vi "NIIE_Undo_Replay Data from History.vi"(8 "Error":errorcluster, 10 "Data":string[](array[string]), 11 "Data":T1={"Class"={"Ants"=refnum, "Layer"=refnum, "Templates"=refnum, "Icon"=refnum, "Glyph"=refnum, "Settings"=refnum, "Tools"=refnum}, "Ref"={"Add Layer"=refnum, "Remove Layer"=refnum, "Line Text"=[], "Body Text Spec"=refnum, "DNL_Font"=refnum, "glyph path str"=refnum, "templates path str"=refnum, "Arrow Up"=refnum, "Arrow Down"=refnum, "IE VI Ref"=refnum, "Glyphs tree"=refnum, "Templates tree"=refnum, "Layer Icon Text"=refnum, "Layer Template"=refnum, "Clipboard"=refnum, "BW icon in"=refnum, "Color icon in"=refnum, "Layer Clust"=refnum, "Body Text"=refnum, "DNL_Framework Templates"=refnum, "Search Templates"=refnum, "TextMarker"=refnum, "Tab Control"=refnum, "Search Glyphs"=refnum, "Line Color"=refnum, "DNL_Glyphs []"=refnum, "Fill Color"=refnum, "Tools"=refnum, "Glyphs tree"=refnum, "Icon"=refnum, "Preview"=refnum, "Ants"=refnum, "Terminals"=refnum, "menu reference"=refnum, "LayerNames"=[], "GlyphLoadAnimation"=refnum, "TemplateLoadAnimation"=refnum, "refreshGlyphs"=refnum, "refreshTemplates"=refnum}, "Support"={"AntsRect"={"left"=0, "top"=0, "right"=0, "bottom"=0}, "Mouse Move Coords"={"Horizontal"=0, "Vertical"=0}, "Mouse Down Coords"={"Horizontal"=0, "Vertical"=0}, "Temp Coord"={"Horizontal"=0, "Vertical"=0}, "Action"=enum."Default", "Edge Color"=4914962, "Fill Color"=16860, "Mouse Down?"=FALSE, "Draft Mode?"=FALSE, "Temp Icon"=bytes[3102], "CTRL Pressed"=FALSE, "Move Selection?"=FALSE, "AntsRect Orig"={"left"=0, "top"=0, "right"=0, "bottom"=0}, "Text"="", "TM Set?"=FALSE, "Mouse inside icon?"=FALSE, "Tool (old value)"=0, "Pencil Move Color"=0, "Swap Colors?"=FALSE, "Shift pressed?"=FALSE}}) -> (0 "Error Out":errorcluster, 3 "Data Out":T1={"Class"={"Ants"=refnum, "Layer"=refnum, "Templates"=refnum, "Icon"=refnum, "Glyph"=refnum, "Settings"=refnum, "Tools"=refnum}, "Ref"={"Add Layer"=refnum, "Remove Layer"=refnum, "Line Text"=[], "Body Text Spec"=refnum, "DNL_Font"=refnum, "glyph path str"=refnum, "templates path str"=refnum, "Arrow Up"=refnum, "Arrow Down"=refnum, "IE VI Ref"=refnum, "Glyphs tree"=refnum, "Templates tree"=refnum, "Layer Icon Text"=refnum, "Layer Template"=refnum, "Clipboard"=refnum, "BW icon in"=refnum, "Color icon in"=refnum, "Layer Clust"=refnum, "Body Text"=refnum, "DNL_Framework Templates"=refnum, "Search Templates"=refnum, "TextMarker"=refnum, "Tab Control"=refnum, "Search Glyphs"=refnum, "Line Color"=refnum, "DNL_Glyphs []"=refnum, "Fill Color"=refnum, "Tools"=refnum, "Glyphs tree"=refnum, "Icon"=refnum, "Preview"=refnum, "Ants"=refnum, "Terminals"=refnum, "menu reference"=refnum, "LayerNames"=[], "GlyphLoadAnimation"=refnum, "TemplateLoadAnimation"=refnum, "refreshGlyphs"=refnum, "refreshTemplates"=refnum}, "Support"={"AntsRect"={"left"=0, "top"=0, "right"=0, "bottom"=0}, "Mouse Move Coords"={"Horizontal"=0, "Vertical"=0}, "Mouse Down Coords"={"Horizontal"=0, "Vertical"=0}, "Temp Coord"={"Horizontal"=0, "Vertical"=0}, "Action"=enum."Default", "Edge Color"=4914962, "Fill Color"=16860, "Mouse Down?"=FALSE, "Draft Mode?"=FALSE, "Temp Icon"=bytes[3102], "CTRL Pressed"=FALSE, "Move Selection?"=FALSE, "AntsRect Orig"={"left"=0, "top"=0, "right"=0, "bottom"=0}, "Text"="", "TM Set?"=FALSE, "Mouse inside icon?"=FALSE, "Tool (old value)"=0, "Pencil Move Color"=0, "Swap Colors?"=FALSE, "Shift pressed?"=FALSE}})   [LabVIEW 2021]
uses:
  Controls/IE Data.ctl
  Class/Ants/Ants.lvclass
  Class/FakedArray/FakedArray.lvclass
  vi.lib/LabVIEW Icon API/lv_icon/Classes/Icon/Icon.lvclass
  Class/Icon Library/Glyph.lvclass
  Class/Settings/Settings.lvclass
  Class/Tools/Tools Paint.lvclass
  Controls/IE Classes.ctl
  Controls/References Cluster.ctl
  Controls/SupportClass.ctl
  <vilib>/Utility/miscctls.llb/LVPoint32TypeDef.ctl
  Controls/ENUM_SupportClass_Action.ctl
  vi.lib/LabVIEW Icon API/lv_icon/Controls/IEColor.ctl
  MB CORE/TypeDefs/Cluster_Layer Data.ctl
  MB CORE/TypeDefs/Cluster_Path&Icon.ctl
  MB CORE/TypeDefs/Cluster_BodyText.ctl
  vi.lib/LabVIEW Icon API/lv_icon/Controls/Font.ctl
  vi.lib/LabVIEW Icon API/lv_icon/Controls/Alignment.ctl
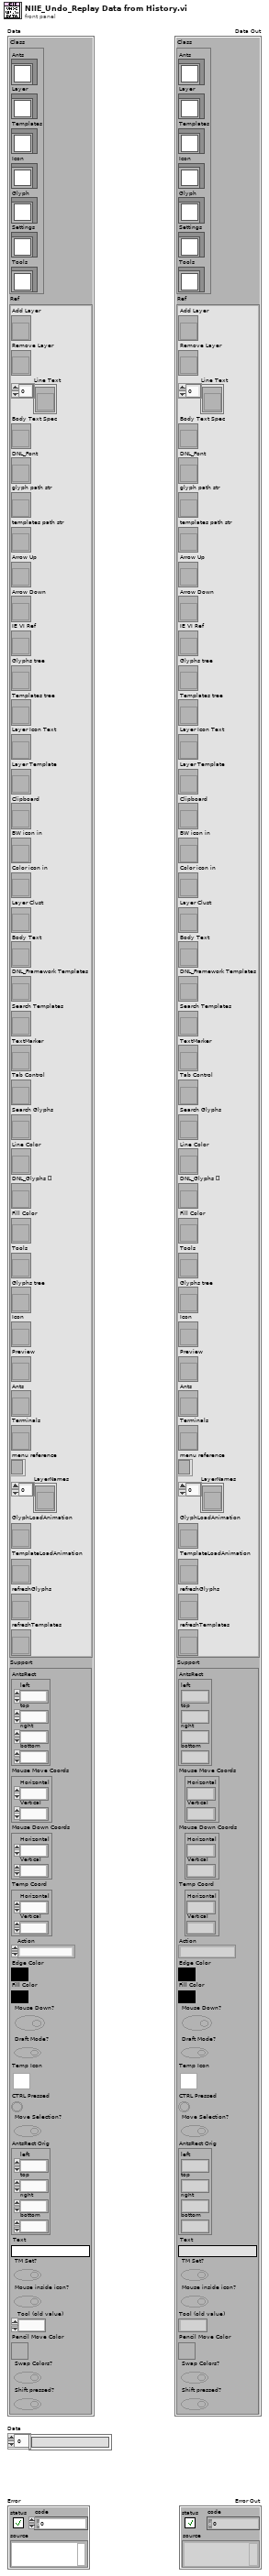
[diagram p1: front panel]
types:
  T1 = typedef "IE Data.ctl" = cluster{"Class":T2, "Ref":T3, "Support":T4}
  T2 = typedef "IE Classes.ctl" = cluster{"Ants":refnum<class "Ants.lvclass">, "Layer":refnum<class "FakedArray.lvclass">, "Templates":refnum<class "FakedArray.lvclass">, "Icon":refnum<class "Icon.lvclass">, "Glyph":refnum<class "Glyph.lvclass">, "Settings":refnum<class "Settings.lvclass">, "Tools":refnum<class "Tools Paint.lvclass">}
  T3 = typedef "References Cluster.ctl" = cluster{"Add Layer":refnum<vi>, "Remove Layer":refnum<vi>, "Line Text":refnum<vi>[], "Body Text Spec":refnum<vi>, "DNL_Font":refnum<vi>, "glyph path str":refnum<vi>, "templates path str":refnum<vi>, "Arrow Up":refnum<vi>, "Arrow Down":refnum<vi>, "IE VI Ref":refnum<vi>, "Glyphs tree":refnum<vi>, "Templates tree":refnum<vi>, "Layer Icon Text":refnum<vi>, "Layer Template":refnum<vi>, "Clipboard":refnum<vi>, "BW icon in":refnum<vi>, "Color icon in":refnum<vi>, "Layer Clust":refnum<vi>, "Body Text":refnum<vi>, "DNL_Framework Templates":refnum<vi>, "Search Templates":refnum<vi>, "TextMarker":refnum<vi>, "Tab Control":refnum<vi>, "Search Glyphs":refnum<vi>, "Line Color":refnum<vi>, "DNL_Glyphs []":refnum<vi>, "Fill Color":refnum<vi>, "Tools":refnum<vi>, "Glyphs tree":refnum<vi>, "Icon":refnum<vi>, "Preview":refnum<vi>, "Ants":refnum<vi>, "Terminals":refnum<vi>, "menu reference":refnum<k9>, "LayerNames":refnum<vi>[], "GlyphLoadAnimation":refnum<vi>, "TemplateLoadAnimation":refnum<vi>, "refreshGlyphs":refnum<vi>, "refreshTemplates":refnum<vi>}
  T4 = typedef "SupportClass.ctl" = cluster{"AntsRect":cluster{"left":i16, "top":i16, "right":i16, "bottom":i16}, "Mouse Move Coords":T5, "Mouse Down Coords":T5, "Temp Coord":T5, "Action":T6, "Edge Color":T7, "Fill Color":T7, "Mouse Down?":bool, "Draft Mode?":bool, "Temp Icon":picture, "CTRL Pressed":bool, "Move Selection?":bool, "AntsRect Orig":cluster{"left":i16, "top":i16, "right":i16, "bottom":i16}, "Text":string, "TM Set?":bool, "Mouse inside icon?":bool, "Tool (old value)":u32, "Pencil Move Color":u32, "Swap Colors?":bool, "Shift pressed?":bool}
  T5 = typedef "LVPoint32TypeDef.ctl" = cluster{"Horizontal":i32, "Vertical":i32}
  T6 = typedef "ENUM_SupportClass_Action.ctl" = enum16{"Default", "Move Selection", "Glyph Library", "Tool"}
  T7 = typedef "IEColor.ctl" = u32
  T8 = typedef "Cluster_BodyText.ctl" = cluster{"Line 1 text":string, "Line 2 text":string, "Line 3 text":string, "Line 4 text":string, "Line 1 color":u32, "Line 2 color":u32, "Line 3 color":u32, "Line 4 color":u32, "Body Text Spec":cluster{"Font":T9, "Alignment":T10, "Size":u8}, "Center text vertically":bool, "Capitalize Text":bool}
  T9 = typedef "Font.ctl" = string
  T10 = typedef "Alignment.ctl" = u16
  T11 = typedef "Cluster_Path&Icon.ctl" = cluster{"Rectangle":cluster{"left":i16, "top":i16, "right":i16, "bottom":i16}, "Path":path, "Image":picture, "Filter":string, "FileName":string}
  T12 = typedef "Cluster_Layer Data.ctl" = cluster{"LayerIcon":picture, "LayerName":string, "Opacity":u8, "Visibility?":bool}
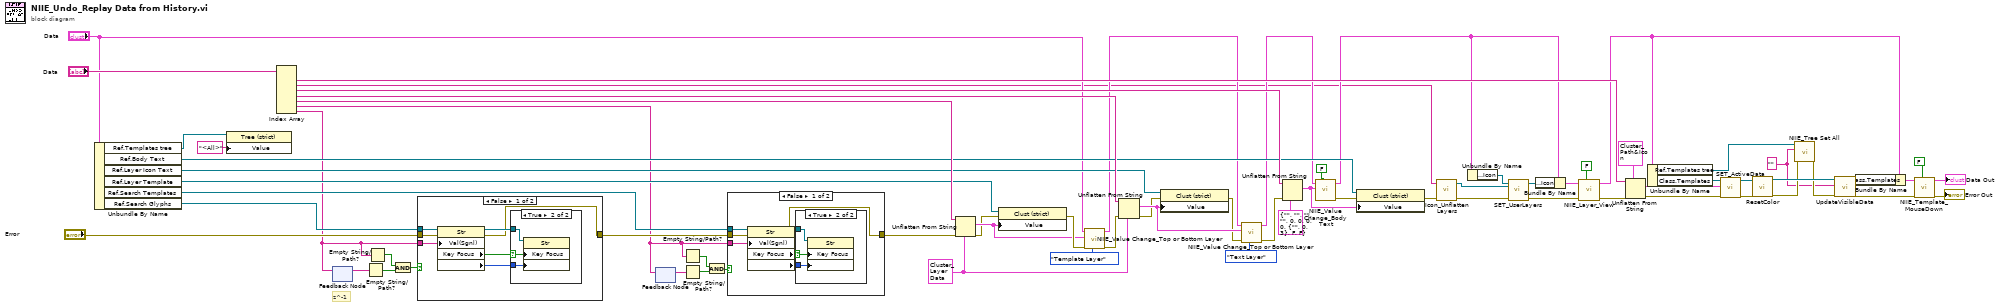
[diagram p0: block diagram]
diagram:
  w1 = "" ("Value")
  w53 = T12 {"LayerIcon"=bytes[3102], "LayerName"="", "Opacity"=100, "Visibility?"=TRUE}
  # "z^-1"
  n1 = Unbundle By Name("Data") -> ("Ref.Templates tree"=w43:refnum<vi>, "Ref.Body Text"=w55:refnum<vi>, "Ref.Layer Icon Text"=w56:refnum<vi>, "Ref.Layer Template"=w57:refnum<vi>, "Ref.Search Templates"=w17:refnum<vi>, "Ref.Search Glyphs"=w19:refnum<vi>)
  n2 = property class="Tree (strict)"(reference=w43, "Value"="<All>") -> ()  [unwired: 1 in, 2 out]
  n3 = Index Array(array="Data") -> (element #1=w60:string, element #2=w20:string, element #3=w70:string, element #4=w71:string, element #5=w72:string, element #6=w7:string, element #7=w11:string)  [unwired: 7 in]
  n4 = feedback-in #1(w11) -> ()
  n5 = feedback #1() -> (w12:string)  [unwired: 1 in]
  n6 = Empty String/Path?(string/path=w12) -> (empty?=w14:bool)
  n7 = Empty String/Path?(string/path=w11) -> (empty?=w9:bool)
  n8 = And(x=w9, y=w14) -> (x .and. y?=w10:bool)
  n9 = case shown="False" w10 {
    tunnel: w11 -> [w79 _]
    tunnel: w19 -> [w78 _]
    tunnel: "Error" -> [w77 w83]
    tunnel: [w73 w83] -> w16
    frame False {
      n10 = property class="Str"(reference=w78, error in=w77, "Val(Sgnl)"=w79) -> (reference out=w74:refnum<vi>, error out=w73:errorcluster, "Key Focus"=w76:bool, "Text.Selection Start"=w75:u32)
      n11 = case shown="True" w76 {
        selector: w76 -> [_ w81]
        tunnel: w75 -> [_ w82]
        tunnel: w74 -> [_ w80]
        frame False {
        }
        frame True {
          n12 = property class="Str"(reference=w80, "Key Focus"=w81, "Text.Selection Start"=w82) -> ()  [unwired: 1 in, 2 out]
        }
      }
    }
    frame True {
    }
  }
  n13 = feedback #2() -> (w8:string)  [unwired: 1 in]
  n14 = feedback-in #2(w7) -> ()
  n15 = Empty String/Path?(string/path=w7) -> (empty?=w5:bool)
  n16 = Empty String/Path?(string/path=w8) -> (empty?=w13:bool)
  n17 = And(x=w5, y=w13) -> (x .and. y?=w6:bool)
  n18 = case shown="False" w6 {
    tunnel: w17 -> [w87 _]
    tunnel: w16 -> [w86 w94]
    tunnel: w7 -> [w85 _]
    tunnel: [w84 w94] -> w15
    frame False {
      n19 = property class="Str"(reference=w87, error in=w86, "Val(Sgnl)"=w85) -> (reference out=w90:refnum<vi>, error out=w84:errorcluster, "Key Focus"=w88:bool, "Text.Selection Start"=w89:u32)
      n20 = case shown="True" w88 {
        selector: w88 -> [_ w92]
        tunnel: w89 -> [_ w93]
        tunnel: w90 -> [_ w91]
        frame False {
        }
        frame True {
          n21 = property class="Str"(reference=w91, "Key Focus"=w92, "Text.Selection Start"=w93) -> ()  [unwired: 1 in, 2 out]
        }
      }
    }
    frame True {
    }
  }
  n22 = Unflatten From String(type=w53, binary string=w72, error in (no error)=w15) -> (value=w49:T12, error out=w39:errorcluster)  [unwired: 3 out]
  n23 = property class="Clust (strict)"(reference=w57, error in=w39, "Value"=w49) -> (error out=w50:errorcluster)  [unwired: 1 out]
  n24 = call "NIIE_Value Change_Top or Bottom Layer.vi"("Type"=enum16{"Template Layer", "Text Layer"}."Template Layer", "Error"=w50, 10:"Data"=w49, 11:"Data"="Data") -> ("Error Out"=w41:errorcluster, "Data Out"=w27:T1)  [unwired: 6 out]
  n25 = Unflatten From String(type=w53, binary string=w71, error in (no error)=w41) -> (value=w47:T12, error out=w40:errorcluster)  [unwired: 3 out]
  n26 = property class="Clust (strict)"(reference=w56, error in=w40, "Value"=w47) -> (error out=w46:errorcluster)  [unwired: 1 out]
  n27 = call "NIIE_Value Change_Top or Bottom Layer.vi"("Type"=enum16{"Template Layer", "Text Layer"}."Text Layer", "Error"=w46, 10:"Data"=w47, 11:"Data"=w27) -> ("Error Out"=w45:errorcluster, "Data Out"=w25:T1)  [unwired: 6 out]
  n28 = Unflatten From String(type=T8 {"Line 1 text"="", "Line 2 text"="", "Line 3 text"="", "Line 4 text"="", "Line 1 color"=0, "Line 2 color"=0, "Line 3 color"=0, "Line 4 color"=0, "Body Text Spec"={"Font"="", "Alignment"=0, "Size"=3}, "Center text vertically"=FALSE, "Capitalize Text"=FALSE} ("Body Text 2"), binary string=w70, error in (no error)=w45) -> (value=w68:T8)  [unwired: 1 in, 3 out]
  n29 = call "NIIE_Value Change_Body Text.vi"("Add To Undo?"=FALSE ("Add to Undo?"), "NewVal"=w68, "Data"=w25) -> ("Error Out"=w66:errorcluster, "Data Out"=w24:T1)  [unwired: 2 in, 5 out]
  n30 = property class="Clust (strict)"(reference=w55, error in=w66, "Value"=w68) -> (error out=w23:errorcluster)  [unwired: 1 out]
  n31 = call "Icon_Unflatten Layers.vi"("Error"=w23, "String"=w20) -> ("Error Out"=w22:errorcluster, "Layers Out"=w21:refnum<class "Layer.lvclass">[])  [unwired: 8 in]
  n32 = Unbundle By Name(w24) -> ("Class.Icon"=w38:refnum<class "Icon.lvclass">)
  n33 = call-dynamic "SET_UserLayers.vi"("error in (no error)"=w22, "Layers"=w21, "Icon.lvclass in"=w38) -> ("error out"=w30:errorcluster, "Icon.lvclass out"=w37:refnum<class "Icon.lvclass">)  [unwired: 7 in]
  n34 = Bundle By Name(cluster=w24, "Class.Icon"=w37) -> (w36:T1)
  n35 = call "NIIE_Layer_View.vi"("Add To Undo?"=FALSE ("Add to Undo?"), "Error"=w30, "Data"=w36) -> ("Error Out"=w54:errorcluster, "Data Out"=w26:T1)  [unwired: 1 in, 6 out]
  n36 = Unflatten From String(type=T11 {"Rectangle"={"left"=0, "top"=0, "right"=0, "bottom"=0}, "Path"=path "", "Image"=bytes[0], "Filter"="", "FileName"=""}, binary string=w60, error in (no error)=w54) -> (value=w64:T11, error out=w35:errorcluster)  [unwired: 3 out]
  n37 = Unbundle By Name(w26) -> ("Ref.Templates tree"=w4:refnum<vi>, "Class.Templates"=w34:refnum<class "FakedArray.lvclass">)
  n38 = call-dynamic "SET_ActiveData.vi"("error in (no error)"=w35, "Active Data"=w64, "FakedArray.lvclass in"=w34) -> ("error out"=w62:errorcluster, "FakedArray.lvclass out"=w61:refnum<class "FakedArray.lvclass">)  [unwired: 7 out]
  n39 = call "ResetColor.vi"("error in (no error)"=w62, "FakedArray in"=w61) -> ("error out"=w3:errorcluster, "FakedArray out"=w63:refnum<class "FakedArray.lvclass">)  [unwired: 8 out]
  n40 = call "NIIE_Tree Set All.vi"("Error"=w3, "Value"=w1, "TreeControl"=w4) -> ("Error Out"=w2:errorcluster)  [unwired: 7 in, 1 out]
  n41 = call-dynamic "UpdateVisibleData.vi"("Error"=w2, "Keyword"=w1, "FakedArray"=w63) -> ("Error Out"=w29:errorcluster, "FakedArray Out"=w33:refnum<class "FakedArray.lvclass">)  [unwired: 2 in, 5 out]
  n42 = Bundle By Name(cluster=w26, "Class.Templates"=w33) -> (w32:T1)
  n43 = call "NIIE_Template_MouseDown.vi"("Add To Undo?"=FALSE ("Add to Undo?"), "Error"=w29, "Data"=w32) -> ("Error Out"=→"Error Out":errorcluster, "Data Out"=→"Data Out":T1)  [unwired: 2 in, 5 out]
